vi "DAC Init Results.vi"(8 "error in":errorcluster, 9 "Log Details?":bool, 10 "tdms file":refnum<k34>, 11 "DAC Inverter in":refnum<class "DAC Inverter.lvclass">) -> (0 "error out":errorcluster, 2 "tdms file out":refnum<k34>)   [LabVIEW 2019, in "DAC.lvlib" / "DAC Inverter.lvclass"]
uses:
  DAC Inverter.lvclass
  DAC.lvclass
  C:/Users/wg/Documents/LV_Projects/test-stand/App/DAC/DAC.lvclass
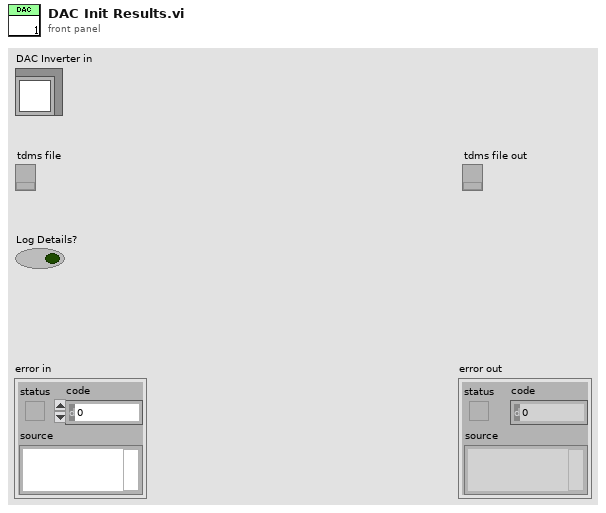
[diagram p1: front panel]
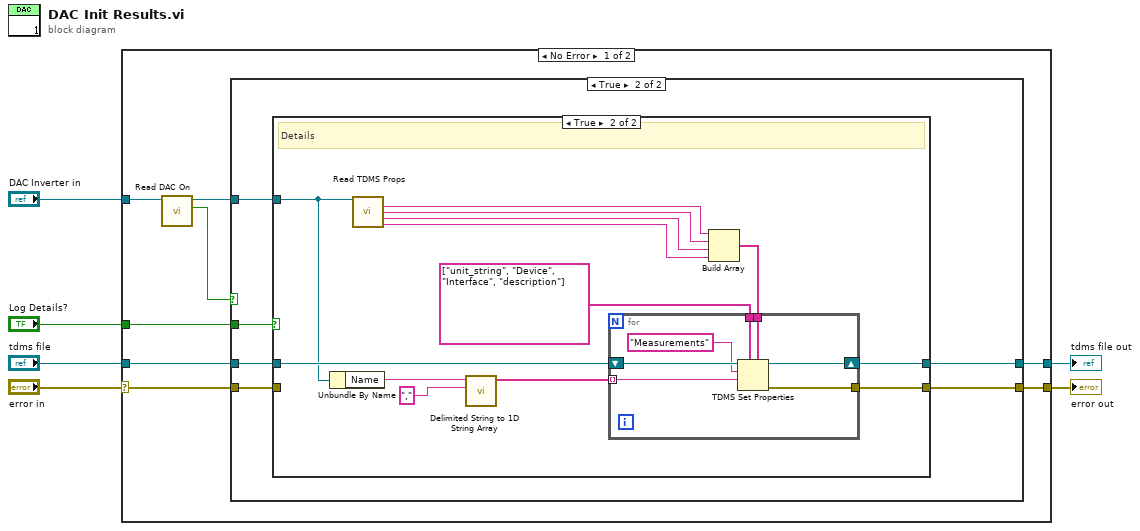
[diagram p0: block diagram]
diagram:
  n1 = case shown="No Error" "error in" {
    selector: "error in" -> [w9 w46]
    tunnel: [w12 w46] -> w3
    tunnel: "DAC Inverter in" -> [w11 _]
    tunnel: "tdms file" -> [w14 w45]
    tunnel: [w13 w45] -> w2
    tunnel: "Log Details?" -> [w7 _]
    frame No Error {
      n2 = call "Read DAC On.vi"("DAC in"=w11) -> ("DAC On"=w8:bool, "DAC out"=w10:refnum<class "DAC Inverter.lvclass">)  [unwired: 8 in, 1 out]
      n3 = case shown="True" w8 {
        tunnel: w14 -> [w16 w22]
        tunnel: [w16 w21] -> w13
        tunnel: [w15 w20] -> w12
        tunnel: w10 -> [_ w19]
        tunnel: w9 -> [w15 w17]
        tunnel: w7 -> [_ w18]
        frame False {
        }
        frame True {
          n4 = case shown="True" w18 {
            tunnel: w22 -> [w24 w37]
            tunnel: [w24 w36] -> w21
            tunnel: [w23 w35] -> w20
            tunnel: w19 -> [_ w29]
            tunnel: w17 -> [w23 _]
            frame False {
            }
            frame True {
              # "Details"
              n5 = Unbundle By Name(w29) -> ("Name"=w32:string)
              n6 = call "Read TDMS Props.vi"("DAC in"=w29) -> ("Result Unit"=w28:string, "DAC Device"=w27:string, "DAC IO"=w26:string, "DAC Description"=w25:string)  [unwired: 10 in, 1 out]
              n7 = call <vilib>:"Delimited String to 1D String Array.vi"("delimiter"=",", "delimited string"=w32) -> ("string array"=w34:string[])  [unwired: 9 in]
              n8 = Build Array(w28, w27, w26, w25) -> (w31:string[])
              n9 = for {
                tunnel: w34 -> [w42] mode=indexing
                tunnel: string[] ["unit_string", "Device", "Interface", "description"] ("property names") -> [w41]
                tunnel: w31 -> [w40]
                tunnel: [w38] -> w35
                shift-right: [w39] -> w36
                shift-left: w37 -> [w44]
                n10 = TDMS Set Properties(5:w40, 7:w41, 9:w42, 10:"Measurements" ("group name in (Untitled)"), 11:w44) -> (0:w38:errorcluster, 3:w39:refnum<k34>)  [unwired: 1 in, 2 out]
              }
            }
          }
        }
      }
    }
    frame Error {
    }
  }
  "error out" <- w3
  "tdms file out" <- w2
